vi "String to Bool.vi"(1 "String":string) -> (0 "Boolean":bool)   [LabVIEW 2026, in "TALOS.lvlib"]
doc: "This VI converts \"0\", \"False\", \"FALSE\" and \"false\" to False, and everything else to True."
uses:
  TALOS.lvlib
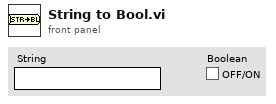
[diagram p1: front panel]
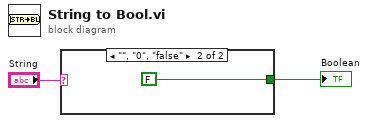
[diagram p0: block diagram]
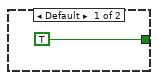
[diagram p2: hidden frame]
diagram:
  n1 = case shown="\"\", \"0\", \"false\"" "String" {
    tunnel: [TRUE FALSE] -> w2
    frame Default {
    }
    frame "", "0", "false" {
    }
  }
  "Boolean" <- w2
